vi "createHeading.vi"(8 "error in (no error)":errorcluster, 9 "Heading Level (-1)":i32=-1, 10 "Heading Text":string, 11 "MS-Word in":refnum<class "MS-Word.lvclass">) -> (0 "error out":errorcluster, 3 "MS-Word out":refnum<class "MS-Word.lvclass">)   [LabVIEW 2017]
doc: "Appends <b>Heading Text</b> with special paragraph style depending on the <b>Heading Level</b> to the Document.\n<b>Heading Level</b>:\n - 1 (default) : body text styling.\n + 0 : document main title.\n + 1 : document sub-titles.\n + 2 : primary paragraph titles.\n + 3 : secondary paragraph titles."
uses:
  Styles/Title/Title.lvclass
  Styles/Heading 1/Heading 1.lvclass
  Styles/Heading 2/Heading 2.lvclass
  Styles/Heading 3/Heading 3.lvclass
  Styles/Style/Style.lvclass
  C:/Users/Neo/Desktop/Dev_Tools_BR/LabVIEW_NPOI/src/Styles/Style/Style.lvclass
  MS-Word.lvclass
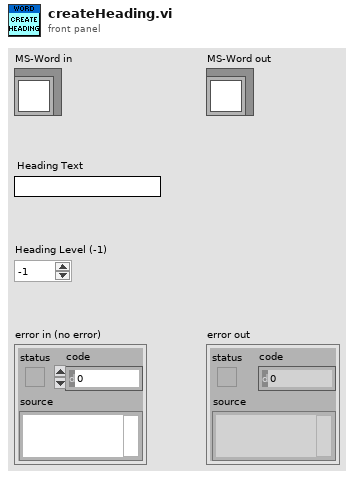
[diagram p1: front panel]
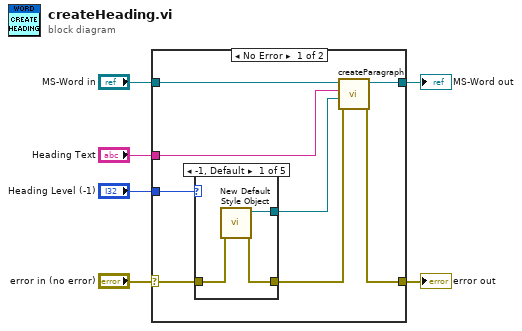
[diagram p0: block diagram]
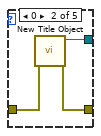
[diagram p2: hidden frame]
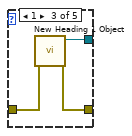
[diagram p3: hidden frame]
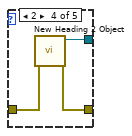
[diagram p4: hidden frame]
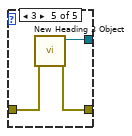
[diagram p5: hidden frame]
diagram:
  n1 = case shown="No Error" "error in (no error)" {
    selector: "error in (no error)" -> [w10 w31]
    tunnel: [w11 w31] -> w5
    tunnel: [w13 w30] -> w3
    tunnel: "MS-Word in" -> [w14 w30]
    tunnel: "Heading Text" -> [w12 _]
    tunnel: "Heading Level (-1)" -> [w9 _]
    frame No Error {
      n2 = case shown="-1, Default" w9 {
        tunnel: w10 -> [w17 w20 w23 w26 w29]
        tunnel: [w16 w19 w22 w25 w28] -> w8
        tunnel: [w15 w18 w21 w24 w27] -> w7
        frame -1, Default {
          n3 = call "New Default Style Object.vi"("error in (no error)"=w17) -> ("error out"=w16:errorcluster, "Style out"=w15:refnum<class "Style.lvclass">)  [unwired: 9 in]
        }
        frame 0 {
          n4 = call "New Title Object.vi"("error in (no error)"=w20) -> ("error out"=w19:errorcluster, "Title out"=w18:refnum<class "Title.lvclass">)  [unwired: 9 in]
        }
        frame 1 {
          n5 = call "New Heading 1 Object.vi"("error in (no error)"=w23) -> ("error out"=w22:errorcluster, "Heading 1 out"=w21:refnum<class "Heading 1.lvclass">)  [unwired: 9 in]
        }
        frame 2 {
          n6 = call "New Heading 2 Object.vi"("error in (no error)"=w26) -> ("error out"=w25:errorcluster, "Heading 2 out"=w24:refnum<class "Heading 2.lvclass">)  [unwired: 9 in]
        }
        frame 3 {
          n7 = call "New Heading 3 Object.vi"("error in (no error)"=w29) -> ("error out"=w28:errorcluster, "Heading 3 out"=w27:refnum<class "Heading 3.lvclass">)  [unwired: 9 in]
        }
      }
      n8 = call-dynamic "createParagraph.vi"("error in (no error)"=w8, "Style"=w7, "Text"=w12, "MS-Word in"=w14) -> ("error out"=w11:errorcluster, "MS-Word out"=w13:refnum<class "MS-Word.lvclass">)  [unwired: 6 in]
    }
    frame Error {
    }
  }
  "error out" <- w5
  "MS-Word out" <- w3
